vi "DualMotorControl_v1.vi"() -> ()   [LabVIEW 2019]
uses:
  <vilib>/myRIO/Common/Instrument Driver Framework/myRIO v1.0/Encoder/typedefs/Encoder Signal Mode.ctl
  <vilib>/myRIO/Instrument Drivers/Onboard IO/Encoder/typedefs/Encoder Reference.ctl
  <vilib>/myRIO/Common/Instrument Driver Framework/Utilities/typedefs/myRIO Generic Hardware Reference.ctl
  <vilib>/myRIO/Common/Instrument Driver Framework/Utilities/typedefs/Hardware Version Enum.ctl
  <vilib>/myRIO/Common/Instrument Driver Framework/Utilities/typedefs/myRIO v1.0 Reference.ctl
  <vilib>/myRIO/Common/Instrument Driver Framework/Utilities/typedefs/Generic FPGA Reference.ctl
  <vilib>/myRIO/Common/Instrument Driver Framework/myRIO v1.0/Encoder/typedefs/Encoder Channels Enum.ctl
  <vilib>/myRIO/Common/Instrument Driver Framework/myRIO v1.0/Encoder/typedefs/Encoder Configuration v1.0.ctl
  <vilib>/userDefined/High Color/nirio_resource_hc.ctl
  <vilib>/Platform/TimedLoop/XDataNode/timing_clust.ctl
  <vilib>/Platform/TimedLoop/XDataNode/nitl_modes.ctl
  <vilib>/Platform/TimedLoop/XDataNode/wakeup.ctl
  <vilib>/myRIO/Instrument Drivers/Onboard IO/PWM/typedefs/PWM Reference.ctl
  <vilib>/myRIO/Common/Instrument Driver Framework/myRIO v1.0/PWM/typedefs/PWM Channels Enum.ctl
  <vilib>/myRIO/Instrument Drivers/Onboard IO/PWM/typedefs/PWM Configuration.ctl
  <vilib>/myRIO/Instrument Drivers/Onboard IO/DIO/typedefs/DIO Reference.ctl
  <vilib>/myRIO/Common/Instrument Driver Framework/myRIO v1.0/DIO/typedefs/DIO Channels List.ctl
  <vilib>/myRIO/Common/Instrument Driver Framework/myRIO v1.0/DIO/typedefs/DIO Channels Enum.ctl
  <vilib>/myRIO/Common/Instrument Driver Framework/Utilities/vis/Is FPGA Ref Available.vi
  <vilib>/myRIO/Common/Instrument Driver Framework/myRIO v1.0/Encoder/vis/myRIO v1.1 Open Encoder.vi
  <vilib>/myRIO/Instrument Drivers/Onboard IO/Encoder/vis/Read.vi
  <vilib>/myRIO/Common/Instrument Driver Framework/myRIO v1.0/PWM/vis/myRIO v1.1 Open PWM.vi
  <vilib>/myRIO/Instrument Drivers/Onboard IO/PWM/vis/Set Duty Cycle and Frequency.vi
  <vilib>/myRIO/Common/Instrument Driver Framework/myRIO v1.0/DIO/vis/myRIO v1.1 Open DIO.vi
  <vilib>/myRIO/Instrument Drivers/Onboard IO/DIO/vis/Write.vi
  <vilib>/myRIO/Common/Instrument Driver Framework/Utilities/vis/Validate Channels.vi
  <vilib>/myRIO/Common/Instrument Driver Framework/myRIO v1.0/Encoder/vis/myRIO v1.0 Reserve Encoder.vi
  <vilib>/myRIO/Common/Instrument Driver Framework/myRIO v1.0/PWM/vis/myRIO v1.0 Reserve PWM.vi
  <vilib>/myRIO/Common/Instrument Driver Framework/myRIO v1.0/DIO/vis/myRIO v1.0 Reserve DIO.vi
  <vilib>/myRIO/Common/Instrument Driver Framework/myRIO v1.0/Encoder/vis/myRIO v1.0 Build MUX Configuration Encoder.vi
  <vilib>/myRIO/Common/Instrument Driver Framework/myRIO v1.0/Resource Manager/vis/myRIO v1.0 Reserve Channel List.vi
  <vilib>/myRIO/Common/Instrument Driver Framework/myRIO v1.0/PWM/vis/myRIO v1.0 Build MUX Configuration PWM.vi
  <vilib>/myRIO/Common/Instrument Driver Framework/myRIO v1.0/DIO/vis/myRIO v1.0 Build MUX Configuration DIO.vi
  <vilib>/myRIO/Common/Instrument Driver Framework/myRIO v1.0/Resource Manager/vis/myRIO v1.0 Create Configuration List.vi
  <vilib>/myRIO/Common/Instrument Driver Framework/myRIO v1.0/Resource Manager/vis/myRIO v1.0 Reserve Channel.vi
  <vilib>/myRIO/Common/Instrument Driver Framework/myRIO v1.0/Resource Manager/vis/myRIO v1.0 Unreserve Channel.vi
  <vilib>/myRIO/Common/Instrument Driver Framework/myRIO v1.0/Resource Manager/vis/myRIO v1.0 Build Mutex Name.vi
  <vilib>/Utility/VariantDataType/GetNumericInfo.vi
  <vilib>/Utility/error.llb/Error Cluster From Error Code.vi
  <vilib>/myRIO/Common/Instrument Driver Framework/myRIO v1.0/myRIO v1.1 Open.vi
  <vilib>/myRIO/Common/Instrument Driver Framework/Utilities/vis/IO Manager.vi
  <vilib>/myRIO/Common/Instrument Driver Framework/Utilities/vis/Configuration Manager.vi
  <vilib>/myRIO/Common/Instrument Driver Framework/myRIO v1.0/Resource Manager/vis/myRIO v1.0 Configure IO.vi
  <vilib>/myRIO/Common/Instrument Driver Framework/myRIO v1.0/myRIO v1.0 Close.vi
  <vilib>/myRIO/Common/Instrument Driver Framework/myRIO v1.0/Encoder/vis/myRIO v1.0 Configure Encoder.vi
  <vilib>/myRIO/Common/Instrument Driver Framework/myRIO v1.0/Encoder/vis/myRIO v1.0 Read Encoder.vi
  <vilib>/Instr/_visa.llb/VISA Configure Serial Port (Instr).vi
  <vilib>/myRIO/Common/Instrument Driver Framework/myRIO v1.0/PWM/vis/myRIO v1.0 Write PWM.vi
  <vilib>/myRIO/Common/Instrument Driver Framework/myRIO v1.0/DIO/vis/myRIO v1.0 Write DIO.vi
  <vilib>/Utility/file.llb/Write Delimited Spreadsheet (DBL).vi
  <vilib>/myRIO/Express VI/Onboard IO/Encoder/Encoder Express VI.xnode
  <vilib>/myRIO/Instrument Drivers/Onboard IO/Encoder/vis/myRIO Encoder Open.xnode
  <vilib>/myRIO/Common/Instrument Driver Framework/myRIO v1.0/Encoder/typedefs/Encoder Count Direction Enum.ctl
  <vilib>/Platform/TimedLoop/XDataNode/XDataNode.xnode
  <vilib>/myRIO/Express VI/Onboard IO/PWM/PWM Express VI.xnode
  <vilib>/myRIO/Instrument Drivers/Onboard IO/PWM/vis/myRIO PWM Open.xnode
  <vilib>/myRIO/Express VI/Onboard IO/DO/DO Express VI.xnode
  <vilib>/myRIO/Instrument Drivers/Onboard IO/DIO/vis/myRIO DIO Open.xnode
  <vilib>/myRIO/Instrument Drivers/Onboard IO/Encoder/Encoder.lvlib
  <vilib>/Platform/TimedLoop/XDataNode/XDNodeRunTimeDep.lvlib
  <vilib>/myRIO/Instrument Drivers/Onboard IO/PWM/PWM.lvlib
  <vilib>/myRIO/Instrument Drivers/Onboard IO/DIO/DIO.lvlib
panel:
  in  "start FIFO":bool=TRUE
  out "Write FIFO error":errorcluster
  out "# elements write":u32=219
  out "timed out?":bool
  out "rt fifo":refnum<k33>
  in  "Buffer factor":dbl=1.5
  out "# elements read":u32
  out "date/time string":string="1970011"
  out "Create FIFO error":errorcluster
  in  "Experiment Mode":string="20250310_servo_sinewave"
  in  "Times":string="0"
  in  "File Path Control":path=path "C:/Rhex_ABAD"
  out "error out":errorcluster
  in  "baud rate (9600)":u32=500000
  in  "VISA resource name":refnum<visa-resource-name>="ASRL2::INSTR"
  in  "stop":bool
  in  "const posotion":dbl=180.0
  out "write to visa":string
  out "read from visa":string
  out "sine position":dbl
  out "time":dbl
  out "iteration":i32
  in  "const(f)/sine(t)":bool
  in  "graph plot freq.":i32=1
  out "Servo Position Graph":cluster{dbl[], dbl[]}[](graph)
  in  "sinewave period":dbl=10.0
  in  "data of 5th order formula\nts,tair,a1-a6":dbl[](array[numeric])
  in  "first or second tripod":bool
  in  "buffer ratio":dbl=0.3
  in  "T_ratio":dbl=10.0
  in  "t_shift":dbl=0.000125
  in  "Encoder_Count":dbl=54991.0
  out "DC Position Chart":cluster{dbl, dbl}(graph)
  in  "Gain":T1={"P Gain"=0.5, "I Gain"=0.0, "D Gain"=0.005}
  in  "Frequency":dbl=1000.0
  out "Duty cycle  2":dbl
  out "Duty cycle":dbl(graph)
  out "DC Velocity Chart":cluster{dbl, dbl}(graph)
  out "DC Position Graph":cluster{dbl[], dbl[]}[](graph)
  out "DC Velocity Graph":cluster{dbl[], dbl[]}[](graph)
  in  "Loop Period":i64=5
  # "Servo motor"
  # "Control botton"
  # "Plot"
  # "visa setting"
  # "servo setting"
  # "Timed loop status"
  # "DC motor"
  # "R-SLIP Parameters"
  # "v = 1; a = 15"
  # "v = 1.25; a = 15"
  # "v = 1.5; a = 15"
  # "0.184067181524967\n0.263820978418769\n256152.551336786\n-30272.30000274\n-9876.03760433421\n-1096.38594197941\n885.91817900106\n-44.6781799901984"
  # "0.215241998794118\n0.254514142390288\n4771.41078363533\n62185.8763006578\n-22508.5336527453\n390.805502041188\n686.695311017595\n-40.4128145310291"
  # "0.163616269216122\n0.27489641502463\n771965.39318528\n-201617.027694185\n8828.08396944145\n-2683.04589908678\n1085.57303422127\n-48.5860395324432"
  # "v = 1.75; a = 15"
  # "v = 2; a = 15"
  # "v = 2.25; a = 15"
  # "0.148651048423414\n0.288542414074344\n1776973.44893281\n-511591.467559457\n38775.9830765103\n-4576.94506688942\n1289.39828252671\n-52.3115561007577"
  # "0.136976185169818\n0.304016701267508\n3461279.85083822\n-993110.73746345\n80544.6579529191\n-6699.48295844177\n1494.82265451498\n-55.8934424469099"
  # "0.134381902205816\n0.369022171779704\n3272804.8365432\n-899365.569589567\n71225.2463409934\n-7039.10791102172\n1512.66147498591\n-59.3408899720725"
  # "FIFO status"
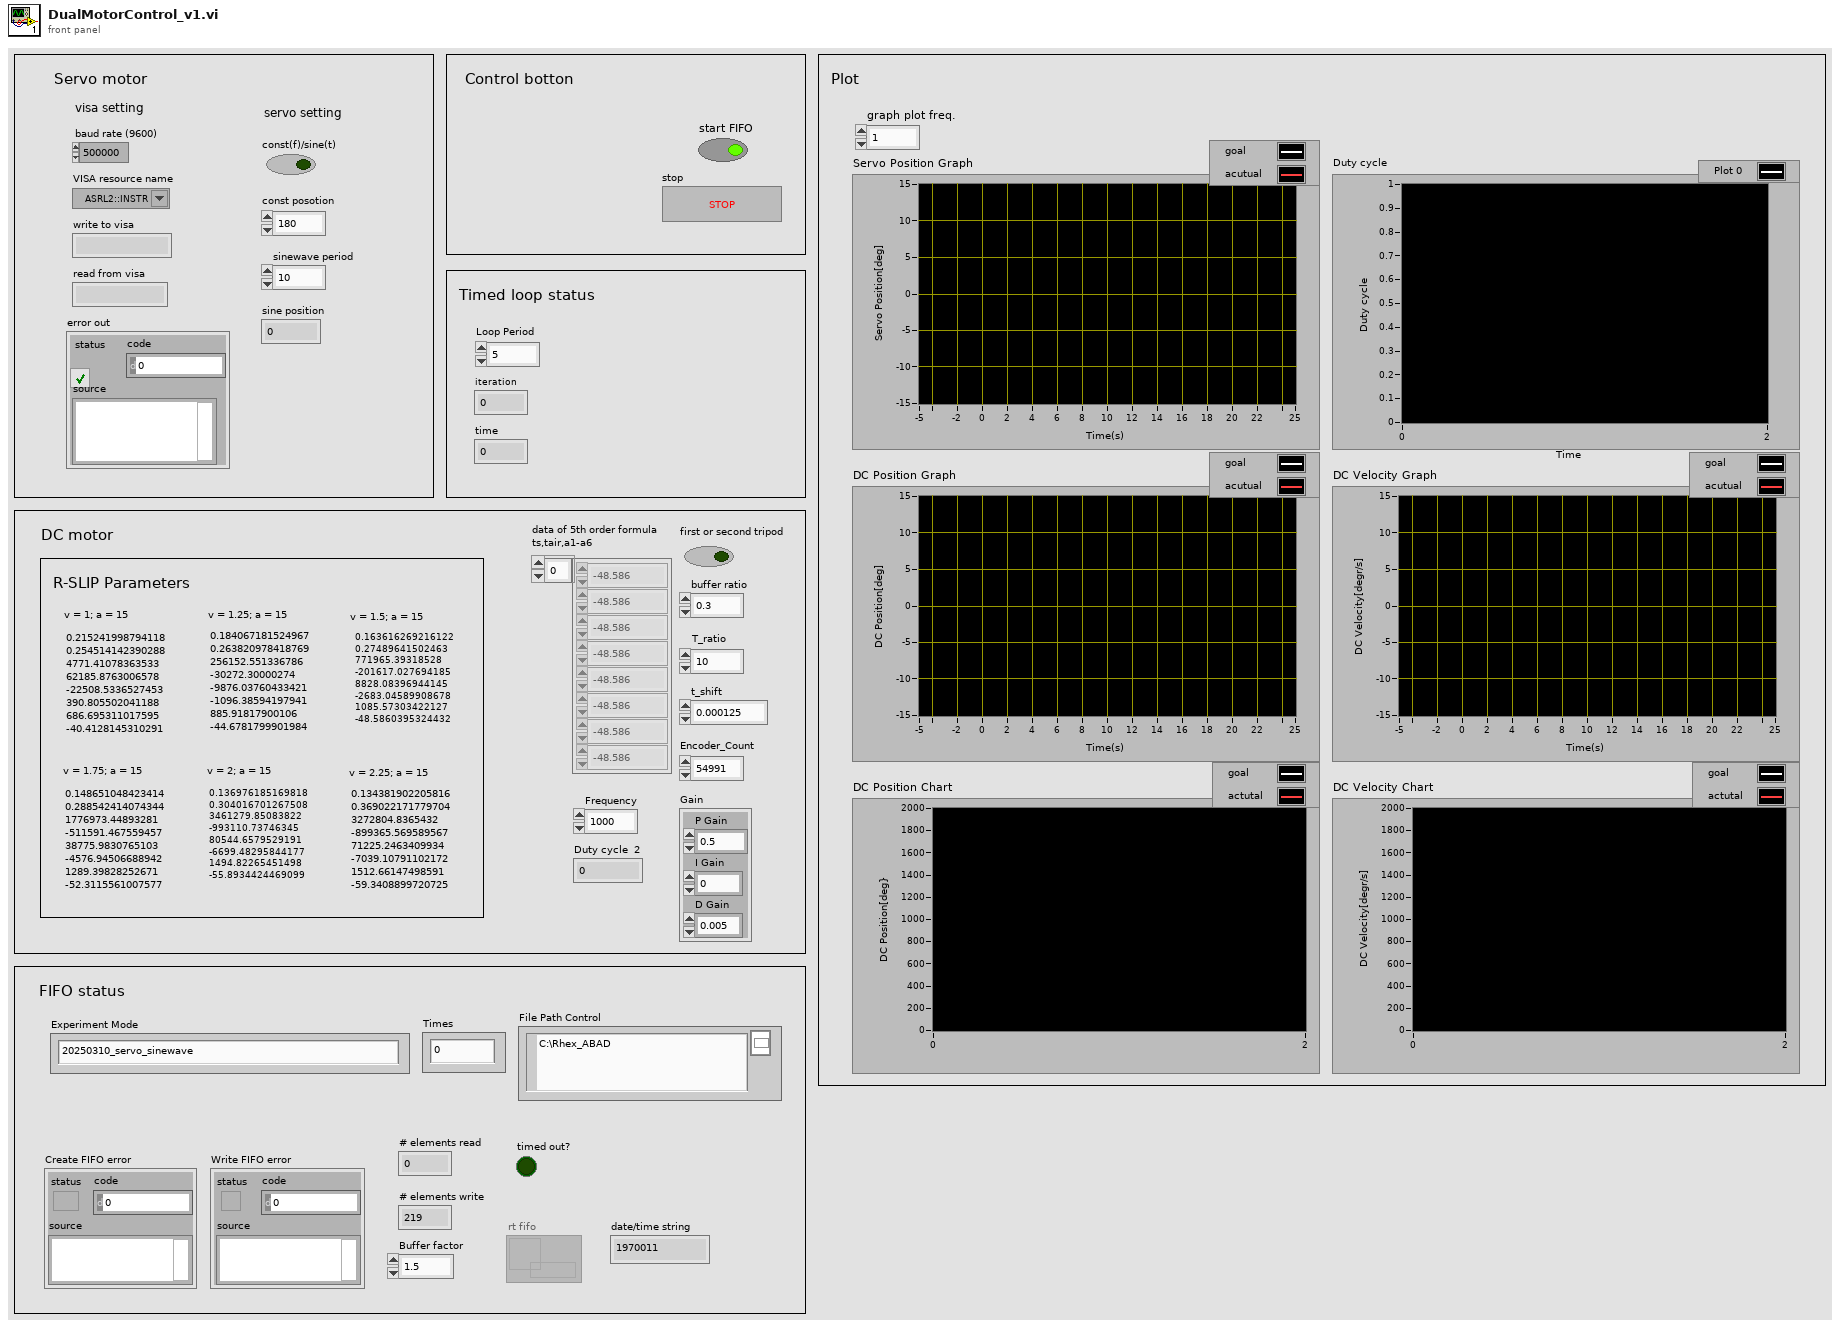
[diagram p1: front panel]
types:
  T1 = cluster{"P Gain":dbl, "I Gain":dbl, "D Gain":dbl}
  T2 = typedef "Encoder.lvlib/Encoder Reference.ctl" = cluster{"myRIO Reference":T3, "Encoder Channels Enum":T7}
  T3 = typedef "myRIO Generic Hardware Reference.ctl" = cluster{"myRIO Model":T4, "myRIO Hardware Reference":T5}
  T4 = typedef "Hardware Version Enum.ctl" = enum16{"Unknown", "myRIO-1900", "myRIO-1950", "roboRIO", "NI ELVIS RIO CM", "ELVIS III"}
  T5 = typedef "myRIO v1.0 Reference.ctl" = cluster{"Generic FPGA Reference":T6, "Allow multiple opens":bool}
  T6 = typedef "Generic FPGA Reference.ctl" = refnum<k20>
  T7 = typedef "Encoder Channels Enum.ctl" = enum16{"Not Connected", "C/ENC0", "C/ENC1", "A/ENC", "A/ENC0", "A/ENC1", "A/ENC2", "A/ENC3", "A/ENC4", "A/ENC5", "A/ENC6", "A/ENC7", "A/ENC8", "A/ENC9", "B/ENC", "B/ENC0", "B/ENC1", "B/ENC2", "B/ENC3", "B/ENC4", "B/ENC5", "B/ENC6", "B/ENC7", "B/ENC8", "B/ENC9", "DIO/ENC0", "DIO/ENC1", "DIO/ENC2", "DIO/ENC3", "DIO/ENC4"}
  T8 = typedef "Encoder Signal Mode.ctl" = enum16{"Quadrature phase signal", "Step and direction signal"}
  T9 = typedef "nirio_resource_hc.ctl" = tag
  T10 = cluster{"set position":dbl, "set position":dbl, "set position":dbl, "set position":dbl, "set position":dbl, "set position":dbl}
  T11 = typedef "DIO.lvlib/DIO Reference.ctl" = cluster{"myRIO Reference":T3, "DIO Channels List":T12}
  T12 = typedef "DIO Channels List.ctl" = T13[]
  T13 = typedef "DIO Channels Enum.ctl" = enum16{"Not Connected", "C/DIO0", "C/DIO1", "C/DIO2", "C/DIO3", "C/DIO4", "C/DIO5", "C/DIO6", "C/DIO7", "A/DIO0", "A/DIO1", "A/DIO2", "A/DIO3", "A/DIO4", "A/DIO5", "A/DIO6", "A/DIO7", "A/DIO8", "A/DIO9", "A/DIO10", "A/DIO11", "A/DIO12", "A/DIO13", "A/DIO14", "A/DIO15", "A/DIO16", "A/DIO17", "A/DIO18", "A/DIO19", "B/DIO0", "B/DIO1", "B/DIO2", "B/DIO3", "B/DIO4", "B/DIO5", "B/DIO6", "B/DIO7", "B/DIO8", "B/DIO9", "B/DIO10", "B/DIO11", "B/DIO12", "B/DIO13", "B/DIO14", "B/DIO15", "B/DIO16", "B/DIO17", "B/DIO18", "B/DIO19", "LED0", "LED1", "LED2", "LED3", "Button0", "DIO/DIO0", "DIO/DIO1", "DIO/DIO2", "DIO/DIO3", "DIO/DIO4", "DIO/DIO5", "DIO/DIO6", "DIO/DIO7", "DIO/DIO8", "DIO/DIO9", "SPI/CS0", "SPI/CS1", "SPI/CS2", "SPI/CS3", "LED RADIO (Green)", "LED RADIO (Red)", "LED COMM (Green)", "LED COMM (Red)", "LED MODE (Green)", "LED MODE (Red)"}
  T14 = typedef "PWM.lvlib/PWM Reference.ctl" = cluster{"myRIO Reference":T3, "PWM Channels Enum":T15, "PWM Configuration":T16}
  T15 = typedef "PWM Channels Enum.ctl" = enum16{"Not Connected", "C/PWM0", "C/PWM1", "A/PWM0", "A/PWM1", "A/PWM2", "A/PWM3", "A/PWM4", "A/PWM5", "A/PWM6", "A/PWM7", "A/PWM8", "A/PWM9", "A/PWM10", "A/PWM11", "A/PWM12", "A/PWM13", "A/PWM14", "A/PWM15", "A/PWM16", "A/PWM17", "A/PWM18", "A/PWM19", "B/PWM0", "B/PWM1", "B/PWM2", "B/PWM3", "B/PWM4", "B/PWM5", "B/PWM6", "B/PWM7", "B/PWM8", "B/PWM9", "B/PWM10", "B/PWM11", "B/PWM12", "B/PWM13", "B/PWM14", "B/PWM15", "B/PWM16", "B/PWM17", "B/PWM18", "B/PWM19", "PWM/PWM0", "PWM/PWM1", "PWM/PWM2", "PWM/PWM3", "PWM/PWM4", "PWM/PWM5", "PWM/PWM6", "PWM/PWM7", "PWM/PWM8", "PWM/PWM9"}
  T16 = typedef "PWM.lvlib/PWM Configuration.ctl" = cluster{"Frequency":dbl, "Duty Cycle":dbl}
  T17 = typedef "XDNodeRunTimeDep.lvlib/timing_clust.ctl" = cluster{"Expected End [f-1]":u64, "Actual End [f-1]":u64, "Finished Late? [f-1]":bool, "Expected End [i-1]":u64, "Actual End [i-1]":u64, "Finished Late? [i-1]":bool, "Expected Start [i]":u64, "Actual Start [i]":u64, "Expected Start [f]":u64, "Actual Start [f]":u64, "Source Name":string, "Structure Name":string, "Period":i64, "Deadline":i64, "Offset":i64, "Start":i64, "Priority":i32, "Timeout":i32, "Mode":T18, "Wakeup Reason":T19, "Error":errorcluster, "Source Type":string, "Secondary Source Type":string, "Global End Time":u64, "Global Start Time":u64, "Frame Duration":u64, "Iteration Duration":u64, "Assigned CPU":i32, "I/O Scan Engine Mode":u32}
  T18 = typedef "XDNodeRunTimeDep.lvlib/nitl_modes.ctl" = enum32{"No Change", "Process missed periods, maintain original phase", "Discard missed periods, maintain original phase", "Process missed periods, ignore original phase", "Discard missed periods, ignore original phase"}
  T19 = typedef "XDNodeRunTimeDep.lvlib/wakeup.ctl" = enum32{"Normal", "Aborted", "Asynchronous wakeup", "Timing source error", "Timed loop error", "Timeout"}
  T20 = cluster{"[0]":dbl, "[1]":dbl, "[2]":dbl, "[3]":dbl, "[4]":dbl, "[5]":dbl}
  T21 = cluster{"set position":i32, "set position":i32, "set position":i32, "set position":i32, "set position":i32, "set position":i32}
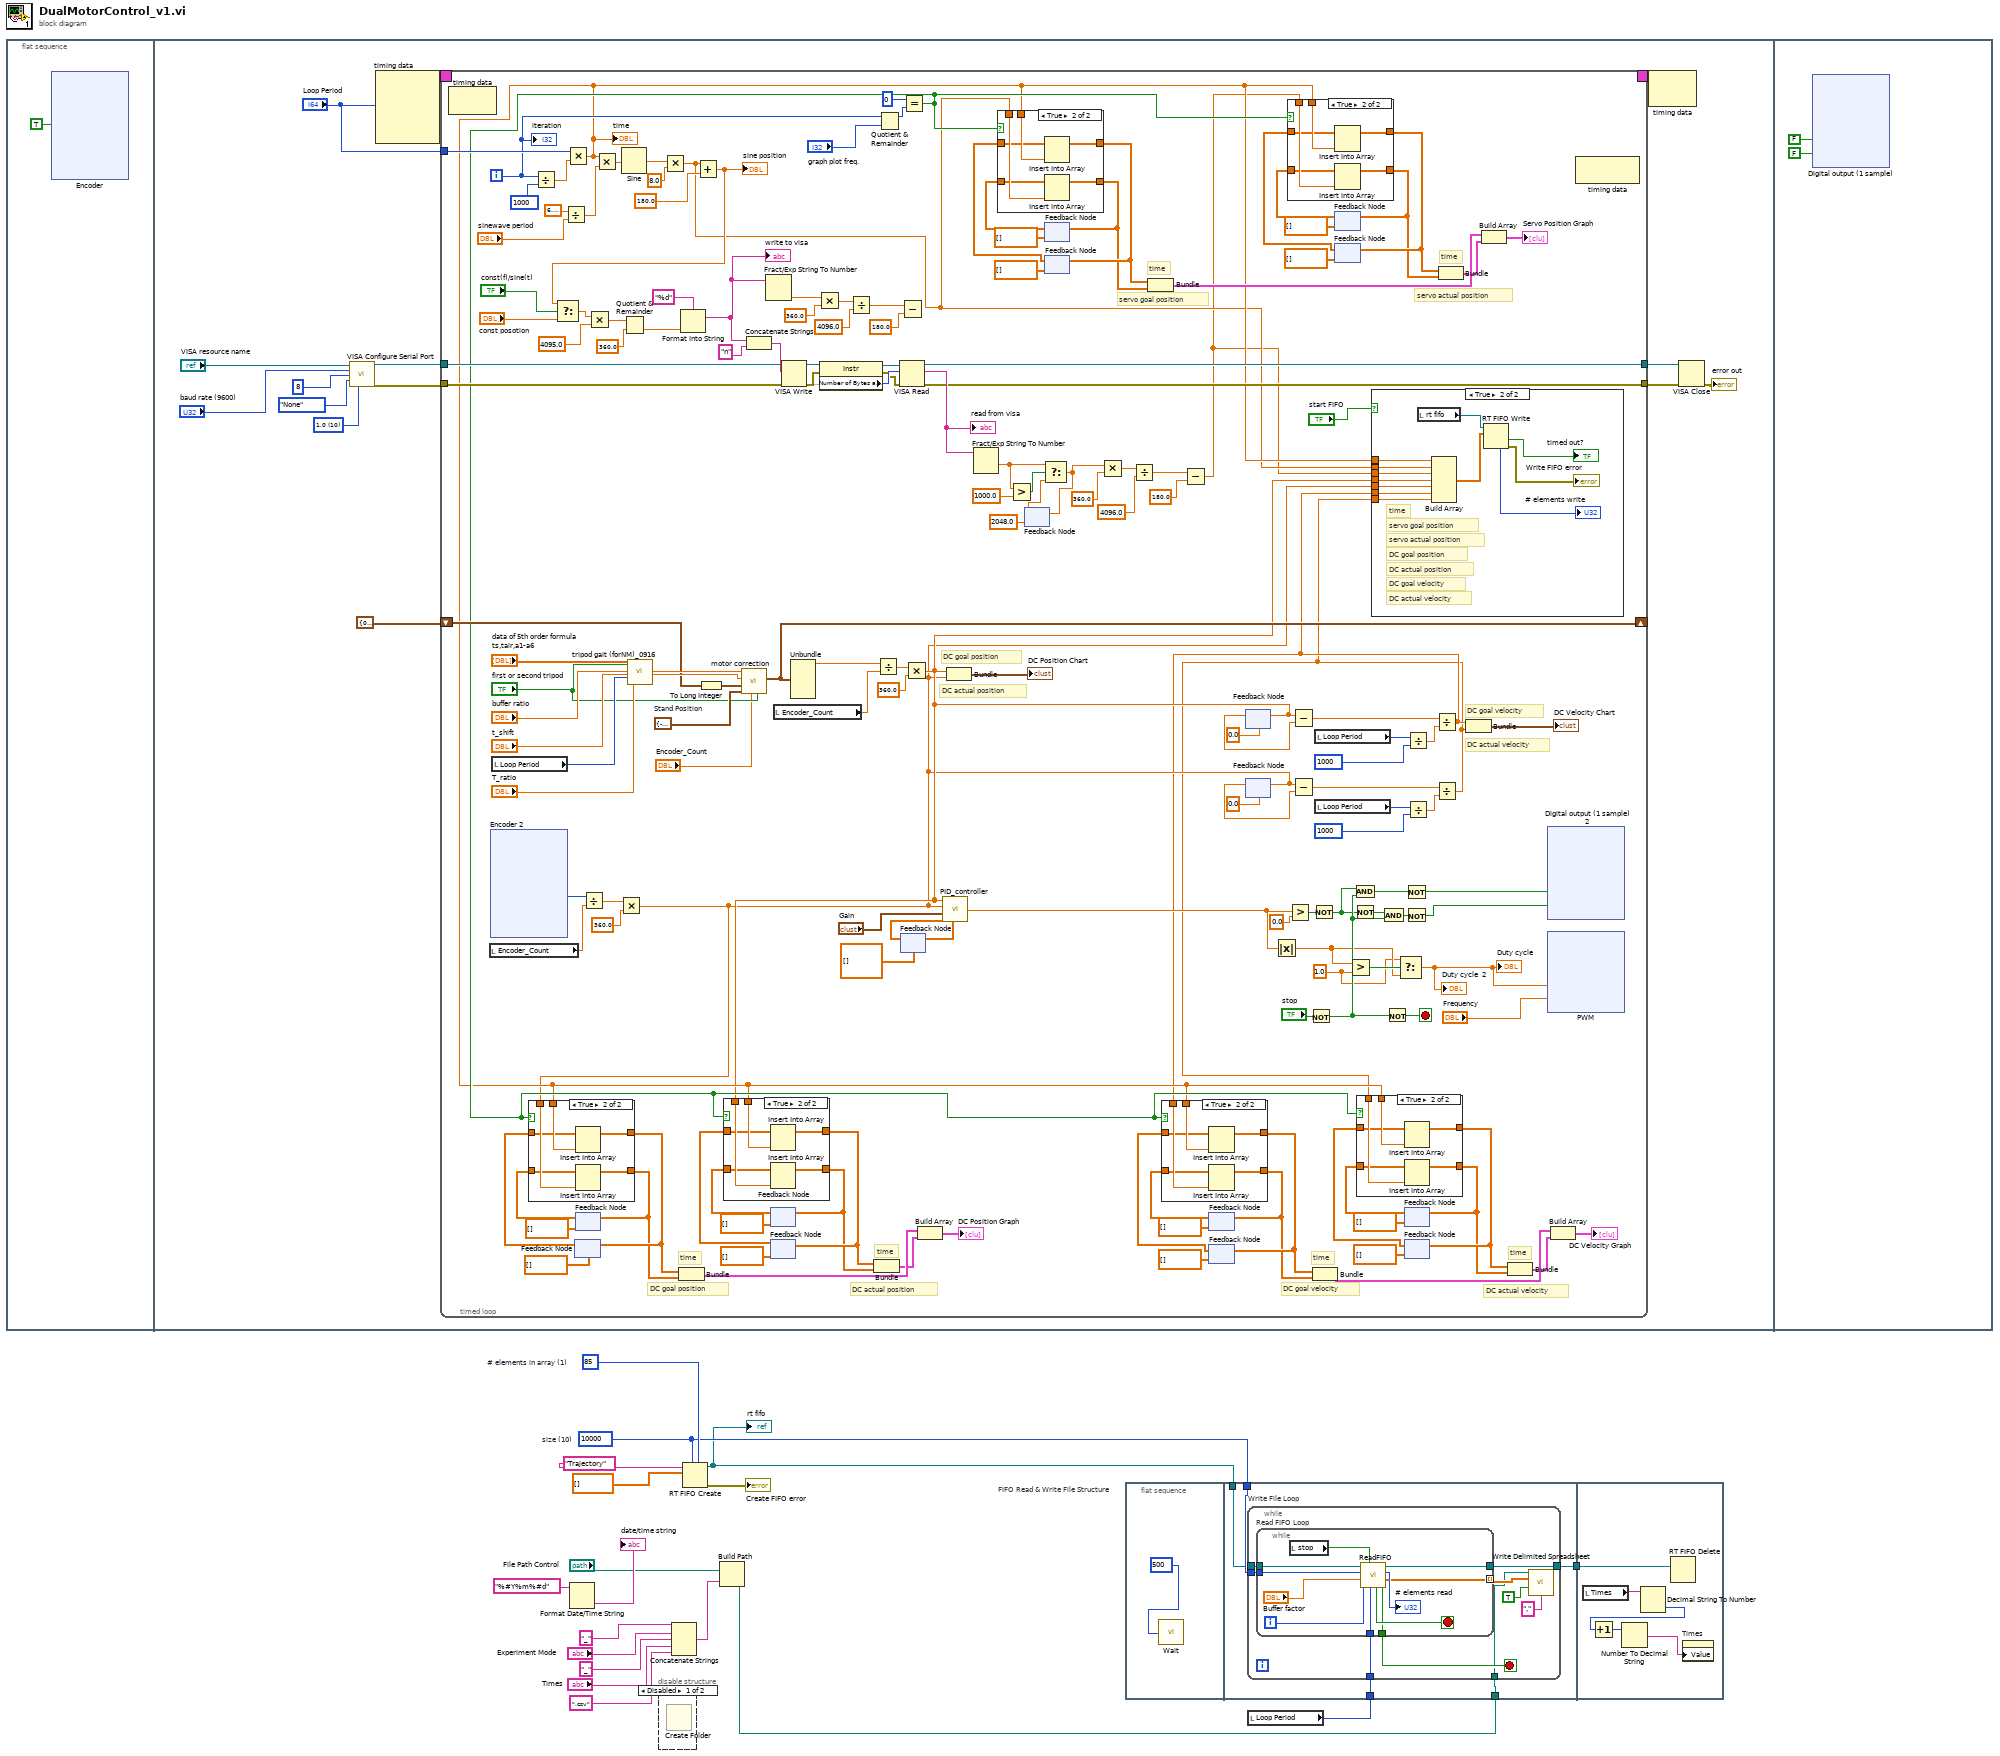
[diagram p0: block diagram]
diagram:
  w7 = u32 85  # # elements in array (1)
  w3 = u32 10000  # size (10)
  n1 = flat-sequence {
    frame #0 {
      n2 = xnode "Encoder"("Reset Counter"=TRUE) -> ()  [unwired: 1 in, 4 out]
    }
    frame #1 {
      w74 = u16 10 items=["1.0"=10, "1.5"=15, "2.0"=20] ("stop bits (10: 1 bit)")
      n3 = call-poly "VISA Configure Serial Port"("VISA resource name"="VISA resource name", "baud rate (9600)"="baud rate (9600)", "data bits (8)"=u16 8, "parity (0:none)"=enum16{"None", "Odd", "Even", "Mark", "Space"}."None", "stop bits (10: 1 bit)"=w74) -> ("VISA resource name out"=w73:refnum<visa-resource-name>, "error out"=w72:errorcluster)  [unwired: 9 in]
      n4 = node-c288("Loop Period") -> (w79:T17)  [unwired: 3 in]
      n5 = timed-loop {
        timing: w79 -> [_]
        timing-out: [_] -> w78
        tunnel: "Loop Period" -> [w189]
        tunnel: w72 -> [w190]
        tunnel: [w187] -> w71
        tunnel: w73 -> [w191]
        tunnel: [w186] -> w67
        shift-right: [w167] -> _
        shift-left: T10 {"set position"=0.0, "set position"=0.0, "set position"=0.0, "set position"=0.0, "set position"=0.0, "set position"=0.0} ("Setpoint_to_motor") -> [w168]
        i -> [w188]
        stop <- w137 stop-if-true
        w134 = 1.0 ("y")
        w166 = T20 {"[0]"=-27495.5, "[1]"=-27495.5, "[2]"=-27495.5, "[3]"=-27495.5, "[4]"=-27495.5, "[5]"=-27495.5}  # Stand Position
        # "time"
        # "DC actual velocity"
        # "time"
        # "DC goal velocity"
        # "time"
        # "DC actual position"
        # "time"
        # "DC goal position"
        # "DC actual velocity"
        # "DC goal velocity"
        # "DC actual position"
        # "DC goal position"
        # "time"
        # "servo actual position"
        # "time"
        # "servo goal position"
        n6 = node-c288() -> ()  [unwired: 1 in, 1 out]
        n7 = local read "Encoder_Count"() -> (w159:dbl)
        n8 = xnode "Encoder 2"() -> ("Counter Value"=w158:i32)  [unwired: 2 in, 3 out]
        n9 = local read "Loop Period"() -> (w173:i64)
        n10 = Divide(x=w188, y=i64 1000) -> (x/y=w221:dbl)
        n11 = Divide(x=6.283185307179586, y="sinewave period") -> (x/y=w177:dbl)
        n12 = Multiply(x=w189, y=w221) -> (x*y=w86:dbl)
        "time" <- w86
        n13 = feedback #1(dbl[] []) -> (w117:dbl[])
        n14 = feedback #2(dbl[] []) -> (w120:dbl[])
        n15 = Divide(x=w158, y=w159) -> (x/y=w156:dbl)
        n16 = Multiply(x=w86, y=w177) -> (x*y=w224:dbl)
        n17 = Multiply(x=w156, y=360.0 ("x")) -> (x*y=w82:dbl)
        n18 = Sine(x=w224) -> (sin(x)=w209:dbl)
        n19 = call "tripod gait (forNM)_0916.vi"("data of 5th order formula\nts,tair,a1-a6"="data of 5th order formula\nts,tair,a1-a6", "first or second"="first or second tripod", "buffer ratio"="buffer ratio", "t_shift"="t_shift", "sample time"=w173, "T_ratio"="T_ratio") -> ("Set Point"=w171:dbl, "Set Point 2"=w170:dbl)  [unwired: 4 in, 16 out]
        n20 = Multiply(x=w209, y=8.0) -> (x*y=w85:dbl)
        n21 = Add(x=w85, y=180.0) -> (x+y=w219:dbl)
        "sine position" <- w219
        n22 = Select(t=w219, s="const(f)/sine(t)", f="const posotion") -> (s? t:f=w217:dbl)
        n23 = Multiply(x=w217, y=4095.0) -> (x*y=w240:dbl)
        n24 = Quotient & Remainder(x=w240, y=360.0) -> (floor(x/y)=w238:dbl)  [unwired: 1 out]
        n25 = Format Into String(format string="%d", w238) -> (resulting string=w231:string)  [unwired: 2 in, 1 out]
        "write to visa" <- w231
        n26 = To Long Integer(number=w168) -> (32bit integer=w169:T21)
        n27 = call "motor correction.vi"("first or second"="first or second tripod", "Encoder_Count"="Encoder_Count", "Stand Position"=w166, "encoder position"=w169, "set position 2"=w170, "set position"=w171) -> ("Setpoint_to_motor"=w167:T10)  [unwired: 4 in, 1 out]
        n28 = Concatenate Strings(w231, "n" ("string")) -> (w242:string)
        n29 = Fract/Exp String To Number(string=w231) -> (number=w230:dbl)  [unwired: 3 in, 1 out]
        n30 = feedback #3(dbl[] []) -> (w116:dbl[])
        n31 = feedback #4(dbl[] []) -> (w113:dbl[])
        n32 = local read "Encoder_Count"() -> (w162:dbl)
        n33 = VISA Write(VISA resource name=w191, write buffer=w242, error in (no error)=w190) -> (VISA resource name out=w207:refnum<visa-resource-name>, error out=w206:errorcluster)  [unwired: 1 out]
        n34 = Unbundle(w167) -> ("set position"=w164:dbl)  [unwired: 5 out]
        n35 = Multiply(x=w230, y=360.0 ("x")) -> (x*y=w228:dbl)
        n36 = property class="Instr"(reference=w207, error in=w206) -> (reference out=w204:refnum<visa-resource-name>, error out=w203:errorcluster, "Serial Settings:Number of Bytes at Serial Port"=w205:u32)
        n37 = Divide(x=w228, y=4096.0) -> (x/y=w233:dbl)
        n38 = Divide(x=w164, y=w162) -> (x/y=w161:dbl)
        n39 = Quotient & Remainder(x=w188, y="graph plot freq.") -> (x-y*floor(x/y)=w212:i32)  [unwired: 1 out]
        n40 = VISA Read(VISA resource name=w204, byte count=w205, error in (no error)=w203) -> (VISA resource name out=w186:refnum<visa-resource-name>, read buffer=w232:string, error out=w187:errorcluster)  [unwired: 1 out]
        "read from visa" <- w232
        n41 = Subtract(x=w233, y=180.0) -> ()  [unwired: 1 out]
        n42 = feedback #5(dbl[] [] ("state(k)")) -> (w153:dbl[])
        n43 = Equal?(x=0, y=w212) -> (x = y?=w88:bool)
        n44 = case shown="True" w88 {
          tunnel: w86 -> [_ w286]
          tunnel: w82 -> [_ w285]
          tunnel: [w280 w284] -> w104
          tunnel: w120 -> [w280 w283]
          tunnel: [w279 w282] -> w105
          tunnel: w117 -> [w279 w281]
          frame False {
          }
          frame True {
            n45 = Insert Into Array(array=w281, new element=w286) -> (w282:dbl[])  [unwired: 1 in]
            n46 = Insert Into Array(array=w283, new element=w285) -> (w284:dbl[])  [unwired: 1 in]
          }
        }
        n47 = feedback-in #1(w105) -> ()
        n48 = feedback-in #2(w104) -> ()
        n49 = Bundle(w105, w104) -> (w112:cluster{dbl[], dbl[]})  [unwired: 1 in]
        n50 = Multiply(x=w161, y=360.0 ("x")) -> (x*y=w83:dbl)
        n51 = case shown="True" w88 {
          tunnel: w86 -> [_ w278]
          tunnel: w83 -> [_ w277]
          tunnel: [w272 w276] -> w108
          tunnel: w116 -> [w272 w275]
          tunnel: [w271 w274] -> w109
          tunnel: w113 -> [w271 w273]
          frame False {
          }
          frame True {
            n52 = Insert Into Array(array=w273, new element=w278) -> (w274:dbl[])  [unwired: 1 in]
            n53 = Insert Into Array(array=w275, new element=w277) -> (w276:dbl[])  [unwired: 1 in]
          }
        }
        n54 = feedback-in #3(w108) -> ()
        n55 = feedback-in #4(w109) -> ()
        n56 = Bundle(w109, w108) -> (w111:cluster{dbl[], dbl[]})  [unwired: 1 in]
        n57 = Build Array(w112, w111) -> (→"DC Position Graph":cluster{dbl[], dbl[]}[])
        n58 = call "PID_controller.vi"("state(k-1)"=w153, "Gain"="Gain", "variable"=w82, "set point"=w83) -> ("PID gain"=w135:dbl, "state(k)"=w152:dbl[])  [unwired: 1 in]
        n59 = feedback-in #5(w152) -> ()
        n60 = Bundle(w83, w82) -> (→"DC Position Chart":cluster{dbl, dbl})  [unwired: 1 in]
        n61 = Fract/Exp String To Number(string=w232) -> (number=w202:dbl)  [unwired: 3 in, 1 out]
        n62 = Greater?(x=w202, y=1000.0) -> (0:w201:bool)
        n63 = feedback #6(2048.0) -> (w181:dbl)
        n64 = Select(t=w202, s=w201, f=w181) -> (s? t:f=w182:dbl)
        n65 = feedback-in #6(w182) -> ()
        n66 = feedback #7(dbl[] []) -> (w216:dbl[])
        n67 = feedback #8(dbl[] []) -> (w213:dbl[])
        n68 = case shown="True" w88 {
          tunnel: w86 -> [_ w419]
          tunnel: w85 -> [_ w418]
          tunnel: [w413 w417] -> w106
          tunnel: w216 -> [w413 w416]
          tunnel: [w412 w415] -> w107
          tunnel: w213 -> [w412 w414]
          frame False {
          }
          frame True {
            n69 = Insert Into Array(array=w414, new element=w419) -> (w415:dbl[])  [unwired: 1 in]
            n70 = Insert Into Array(array=w416, new element=w418) -> (w417:dbl[])  [unwired: 1 in]
          }
        }
        n71 = feedback-in #7(w106) -> ()
        n72 = feedback-in #8(w107) -> ()
        n73 = Multiply(x=w182, y=360.0 ("x")) -> (x*y=w225:dbl)
        n74 = Divide(x=w225, y=4096.0) -> (x/y=w227:dbl)
        n75 = Bundle(w107, w106) -> (w196:cluster{dbl[], dbl[]})  [unwired: 1 in]
        n76 = Subtract(x=w227, y=180.0) -> (x-y=w84:dbl)
        n77 = feedback #9(dbl[] []) -> (w103:dbl[])
        n78 = feedback #10(dbl[] []) -> (w100:dbl[])
        n79 = feedback #11(0.0) -> (w128:dbl)
        n80 = feedback-in #11(w83) -> ()
        n81 = feedback #12(0.0) -> (w122:dbl)
        n82 = feedback-in #12(w82) -> ()
        n83 = Absolute Value(x=w135) -> (abs(x)=w144:dbl)
        n84 = Greater?(x=w135, y=0.0) -> (0:w146:bool)
        n85 = Subtract(x=w83, y=w128) -> (x-y=w131:dbl)
        n86 = Subtract(x=w82, y=w122) -> (x-y=w124:dbl)
        n87 = Not(x="stop") -> (.not. x?=w148:bool)
        n88 = Not(x=w146) -> (.not. x?=w143:bool)
        n89 = local read "Loop Period"() -> (w130:i64)
        n90 = local read "Loop Period"() -> (w121:i64)
        n91 = feedback #13(dbl[] []) -> (w200:dbl[])
        n92 = feedback #14(dbl[] []) -> (w197:dbl[])
        n93 = case shown="True" w88 {
          tunnel: w86 -> [_ w411]
          tunnel: w84 -> [_ w410]
          tunnel: [w405 w409] -> w192
          tunnel: w200 -> [w405 w408]
          tunnel: [w404 w407] -> w193
          tunnel: w197 -> [w404 w406]
          frame False {
          }
          frame True {
            n94 = Insert Into Array(array=w406, new element=w411) -> (w407:dbl[])  [unwired: 1 in]
            n95 = Insert Into Array(array=w408, new element=w410) -> (w409:dbl[])  [unwired: 1 in]
          }
        }
        n96 = feedback-in #13(w192) -> ()
        n97 = feedback-in #14(w193) -> ()
        n98 = Greater?(x=w144, y=w134) -> (0:w145:bool)
        n99 = And(x=w143, y=w148) -> (x .and. y?=w140:bool)
        n100 = Not(x=w143) -> (.not. x?=w149:bool)
        n101 = And(x=w149, y=w148) -> (x .and. y?=w142:bool)
        n102 = Not(x=w148) -> (.not. x?=w137:bool)
        n103 = Select(t=w134, s=w145, f=w144) -> (s? t:f=w138:dbl)
        "Duty cycle  2" <- w138
        "Duty cycle" <- w138
        n104 = Not(x=w140) -> (.not. x?=w139:bool)
        n105 = Not(x=w142) -> (.not. x?=w141:bool)
        n106 = feedback #15(dbl[] []) -> (w99:dbl[])
        n107 = feedback #16(dbl[] []) -> (w96:dbl[])
        n108 = Divide(x=w130, y=i64 1000) -> (x/y=w132:dbl)
        n109 = Divide(x=w121, y=i64 1000) -> (x/y=w125:dbl)
        n110 = Divide(x=w131, y=w132) -> (x/y=w81:dbl)
        n111 = case shown="True" w88 {
          tunnel: w86 -> [_ w270]
          tunnel: w81 -> [_ w269]
          tunnel: [w264 w268] -> w89
          tunnel: w103 -> [w264 w267]
          tunnel: [w263 w266] -> w90
          tunnel: w100 -> [w263 w265]
          frame False {
          }
          frame True {
            n112 = Insert Into Array(array=w265, new element=w270) -> (w266:dbl[])  [unwired: 1 in]
            n113 = Insert Into Array(array=w267, new element=w269) -> (w268:dbl[])  [unwired: 1 in]
          }
        }
        n114 = feedback-in #9(w89) -> ()
        n115 = feedback-in #10(w90) -> ()
        n116 = Bundle(w90, w89) -> (w95:cluster{dbl[], dbl[]})  [unwired: 1 in]
        n117 = Divide(x=w124, y=w125) -> (x/y=w80:dbl)
        n118 = case shown="True" w88 {
          tunnel: w86 -> [_ w262]
          tunnel: w80 -> [_ w261]
          tunnel: [w256 w260] -> w91
          tunnel: w99 -> [w256 w259]
          tunnel: [w255 w258] -> w92
          tunnel: w96 -> [w255 w257]
          frame False {
          }
          frame True {
            n119 = Insert Into Array(array=w257, new element=w262) -> (w258:dbl[])  [unwired: 1 in]
            n120 = Insert Into Array(array=w259, new element=w261) -> (w260:dbl[])  [unwired: 1 in]
          }
        }
        n121 = case shown="True" "start FIFO" {
          tunnel: w86 -> [_ w249]
          tunnel: w85 -> [_ w248]
          tunnel: w84 -> [_ w247]
          tunnel: w83 -> [_ w246]
          tunnel: w82 -> [_ w245]
          tunnel: w81 -> [_ w244]
          tunnel: w80 -> [_ w243]
          frame False {
          }
          frame True {
            # "DC actual velocity"
            # "DC goal velocity"
            # "DC actual position"
            # "DC goal position"
            # "time"
            # "servo actual position"
            # "servo goal position"
            n122 = local read "rt fifo"() -> (w251:refnum<k33>)
            n123 = Build Array(w249, w248, w247, w246, w245, w244, w243) -> (w250:dbl[])
            n124 = RT FIFO Write(0:w251, 1:w250) -> (7:→"# elements write":u32, 10:→"timed out?":bool, 11:→"Write FIFO error":errorcluster)  [unwired: 3 in, 1 out]
          }
        }
        n125 = feedback-in #15(w91) -> ()
        n126 = feedback-in #16(w92) -> ()
        n127 = Bundle(w193, w192) -> (w195:cluster{dbl[], dbl[]})  [unwired: 1 in]
        n128 = Bundle(w81, w80) -> (→"DC Velocity Chart":cluster{dbl, dbl})  [unwired: 1 in]
        n129 = Build Array(w196, w195) -> (→"Servo Position Graph":cluster{dbl[], dbl[]}[])
        n130 = Bundle(w92, w91) -> (w94:cluster{dbl[], dbl[]})  [unwired: 1 in]
        n131 = xnode "Digital output (1 sample) 2"("A/DIO0 (Pin 11)"=w139, "A/DIO1 (Pin 13)"=w141) -> ()  [unwired: 1 in, 1 out]
        n132 = xnode "PWM"("Duty Cycle"=w138, "Frequency [Hz]"="Frequency") -> ()  [unwired: 1 in, 1 out]
        n133 = Build Array(w95, w94) -> (→"DC Velocity Graph":cluster{dbl[], dbl[]}[])
        n134 = node-c288() -> ()  [unwired: 1 in, 1 out]
        "iteration" <- w188
      }
      n135 = node-c288(w78) -> ()  [unwired: 1 out]
      n136 = VISA Close(VISA resource name=w67, error in (no error)=w71) -> (error out=→"error out":errorcluster)
    }
    frame #2 {
      n137 = xnode "Digital output (1 sample)"("A/DIO0 (Pin 11)"=FALSE, "A/DIO1 (Pin 13)"=FALSE) -> ()  [unwired: 1 in, 1 out]
    }
  }
  n138 = Format Date/Time String(time format string (%c)="%#Y%m%#d" ("String 2")) -> (date/time string=→"date/time string":string)  [unwired: 2 in]
  n139 = disable-structure shown="Disabled" {
    frame Disabled {
      n140 = Create Folder() -> ()  [unwired: 3 in, 3 out]
    }
    frame Enabled {
    }
  }
  n141 = Concatenate Strings("_" ("String 2"), "Experiment Mode", "_" ("String 2"), "Times", ".csv" ("string")) -> (w11:string)
  n142 = RT FIFO Create(0:"Trajectory" ("name (unnamed)"), 1:dbl[] [], 4:w3, 6:w7) -> (8:w2:refnum<k33>, 11:→"Create FIFO error":errorcluster)  [unwired: 4 in, 1 out]
  "rt fifo" <- w2
  n143 = Build Path(base path="File Path Control", name or relative path=w11) -> (appended path=w9:path)
  n144 = flat-sequence "FIFO Read & Write File Structure" {
    tunnel: w3 -> [w468]
    tunnel: w1 -> [w467]
    tunnel: w9 -> [w466]
    tunnel: w2 -> [w465]
    tunnel: [w469] -> w18
    tunnel: w18 -> [w490]
    frame #0 {
      n145 = call "Wait"("Count(mSec)"=u32 500 ("Count(uSec)")) -> ()  [unwired: 1 out]
    }
    frame #1 {
      n146 = while "Write File Loop" {
        tunnel: w465 -> [w478]
        tunnel: [w477] -> w469
        tunnel: w468 -> [w476]
        tunnel: w467 -> [w475]
        tunnel: w466 -> [w470]
        stop <- w474 stop-if-true
        n147 = while "Read FIFO Loop" {
          tunnel: w478 -> [w488]
          tunnel: [w482] -> w477
          tunnel: w476 -> [w487]
          tunnel: w475 -> [w485]
          tunnel: [w483] -> w474
          tunnel: [w480] -> w471 mode=indexing
          i -> [w479]
          stop <- w484 stop-if-true
          n148 = local read "stop"() -> (w489:bool)
          n149 = call "ReadFIFO.vi"("dt of Timeloop(ms)"=w485, "Stop"=w489, "Count"=w479, "Buffer factor"="Buffer factor", "FIFO size"=w487, "RT FIFO"=w488) -> ("Stop write file"=w483:bool, "element out"=w480:dbl[], "# elements"=→"# elements read":u32, "RT FIFO (to delete)"=w482:refnum<k33>, "Stop read file"=w484:bool)  [unwired: 1 in]
        }
        n150 = call-poly <vilib>:"Write Delimited Spreadsheet.vi"("file path (dialog if empty)"=w470, "2D data"=w471, "append to file? (new file:F)"=TRUE, "delimiter (\\t)"="," ("delimiter (\\t)")) -> ()  [unwired: 10 in, 2 out]
      }
    }
    frame #2 {
      n151 = local read "Times"() -> (w492:string)
      n152 = Decimal String To Number(string=w492) -> (number=w494:i32)  [unwired: 2 in, 1 out]
      n153 = Increment(x=w494) -> (x+1=w493:i32)
      n154 = Number To Decimal String(number=w493) -> (decimal integer string=w491:string)  [unwired: 1 in]
      n155 = RT FIFO Delete(0:w490) -> ()  [unwired: 2 in, 1 out]
      n156 = property on="Times" class="Str"("Value"=w491) -> ()  [unwired: 2 in, 2 out]
    }
  }
  n157 = local read "Loop Period"() -> (w1:i64)
